vi "FGV_Dither.vi"(5 "Action":enum16{"Set", "Get "}(ring), 7 "Moisture Data In":T1={"Moisture (V)"=2.5, "Dither"=0.1, "Stop"=FALSE}, 11 "Error In":errorcluster) -> (8 "Moisture Data Out":T1={"Moisture (V)"=2.5, "Dither"=0.1, "Stop"=FALSE}, 15 "Error Out":errorcluster)   [LabVIEW 2016]
doc: "This VI gets or sets the GEA2 reference."
uses:
  Controls/Moisture Data.ctl
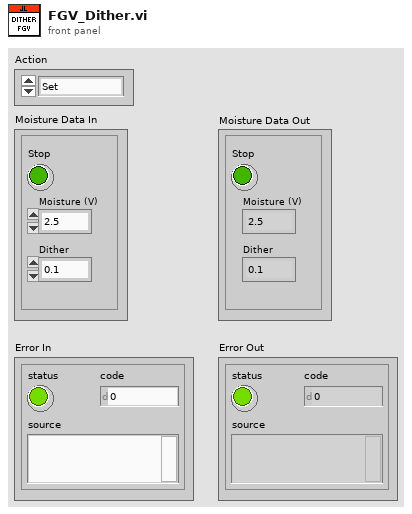
[diagram p1: front panel]
types:
  T1 = typedef "Moisture Data.ctl" = cluster{"Moisture (V)":dbl, "Dither":dbl, "Stop":bool}
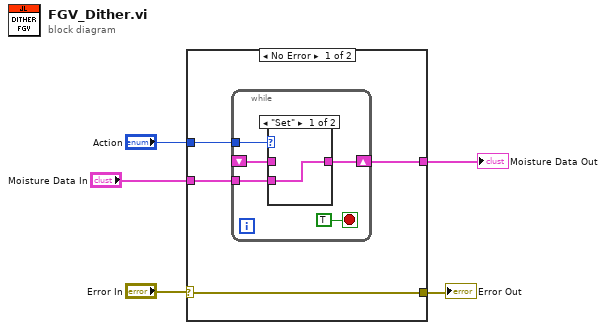
[diagram p0: block diagram]
diagram:
  n1 = case shown="No Error" "Error In" {
    selector: "Error In" -> [w6 w17]
    tunnel: "Action" -> [w9 _]
    tunnel: "Moisture Data In" -> [w8 _]
    tunnel: [w7 _] -> w2
    tunnel: [w6 w17] -> w3
    frame No Error {
      n2 = while {
        tunnel: w9 -> [w13]
        tunnel: w8 -> [w12]
        shift-right: [w11] -> w7
        shift-left: _ -> [w10]
        stop <- TRUE stop-if-true
        n3 = case shown="\"Set\"" w13 {
          tunnel: w12 -> [w15 _]
          tunnel: [w15 w16] -> w11
          tunnel: w10 -> [_ w16]
          frame "Set" {
          }
          frame "Get " {
          }
        }
      }
    }
    frame Error {
    }
  }
  "Error Out" <- w3
  "Moisture Data Out" <- w2
